vi "VideoRecorderOI.vi"() -> ()   [LabVIEW 2011]
uses:
  <instrlib>/niHWS/nihws.llb/niHWS Open File Permissions ID.ctl
  <vilib>/DAQmx/read.llb/DAQmx Read (Analog 1D Wfm NChan NSamp).vi
  <vilib>/DAQmx/create/channels.llb/DAQmx Create Channel (AI-Voltage-Basic).vi
  <vilib>/DAQmx/configure/timing.llb/DAQmx Timing (Sample Clock).vi
  <vilib>/DAQmx/miscellaneous.llb/DAQmx Fill In Error Info.vi
  <instrlib>/niHWS/nihws.llb/niHWS Write Analog WDT.vi
  <instrlib>/niHWS/nihws.llb/niHWS Write Analog DBL.vi
  <vilib>/vision/driver/NI_Vision_Acquisition_Software.lvlib
  C:/Program Files/National Instruments/LabVIEW 2011/resource/objmgr/imaqdx.rc
  <vilib>/ptbypt/NI_PtbyPt.lvlib
  C:/Program Files/National Instruments/LabVIEW 2011/resource/objmgr/daqmx.rc
  <vilib>/vision/NI_Vision_Development_Module.lvlib
panel:
  in  "?":enum32{"Settings", "Monitor"}(tab)
  in  "Phtd":bool=TRUE
  in  "% Quality":i32=-1
  in  "Selected Path for AVI":path
  in  "Compressor":string(combo)="DV Video Encoder"
  in  "Video Modes":string(combo)="1280x1024 RGB8 10.00fps"
  in  "Camera":string(combo)="uc480 Capture Device 1"
  in  "Recording channels":tag
  in  "Channel Names":string[](array[string])
  in  "reduce size":bool
  in  "Downsampling factor":i32=15
  in  "VISA resource name":refnum<visa-resource-name>
  in  "DPI":dbl=3500.0
  in  "Video":bool=TRUE
  in  "Ephys":bool
  in  "Mouse":bool=TRUE
  in  "Start":bool
  out "Eye camera":T1(plugin-control)
  out "Ephys Recoding Signals":waveform(dbl)[](graph)
  out "Activity":dbl(graph)
  in  "stop":bool
  out "Rec Time":dbl format="%#_3g"
  in  "Display":bool
  out "fps":dbl format="%#_2g"
  in  "Rec":bool
  # "File settings"
  # "Ephys Channels"
  # "Camera settings"
  # "Mouse"
  # "On"
  # "Off"
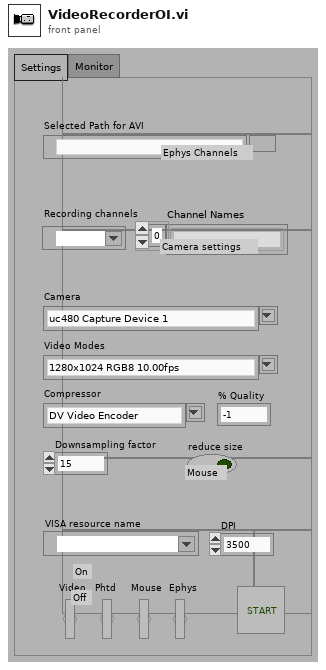
[diagram p1: front panel]
types:
  T1 = typedef "IMAQ Image.ctl" = refnum<image>
  T2 = typedef "niHWS Open File Permissions ID.ctl" = enum32{"Read Only", "Read/Write Existing", "Read/Write/Create New", "Read/Write/Create New Always"}
  T3 = cluster{"Type":u32, "Version":u32, "Flags":u32, "SerialNumberHigh":u32, "SerialNumberLow":u32, "BusType":u32, "InterfaceName":string, "VendorName":string, "ModelName":string, "CameraFileName":string, "CameraAttributeURL":string}[]
  T4 = cluster{"Type":u32, "Version":u32, "Flags":u32, "SerialNumberHigh":u32, "SerialNumberLow":u32, "BusType":u32, "InterfaceName":string, "VendorName":string, "ModelName":string, "CameraFileName":string, "CameraAttributeURL":string}
  T5 = typedef "IMAQdx.ctl" = refnum<k21>
  T6 = cluster{"Video Mode":u32, "Video Mode Name":string}[]
  T7 = typedef "AviRefnum.ctl" = refnum<k1>
  T8 = typedef "Image Type" = u32
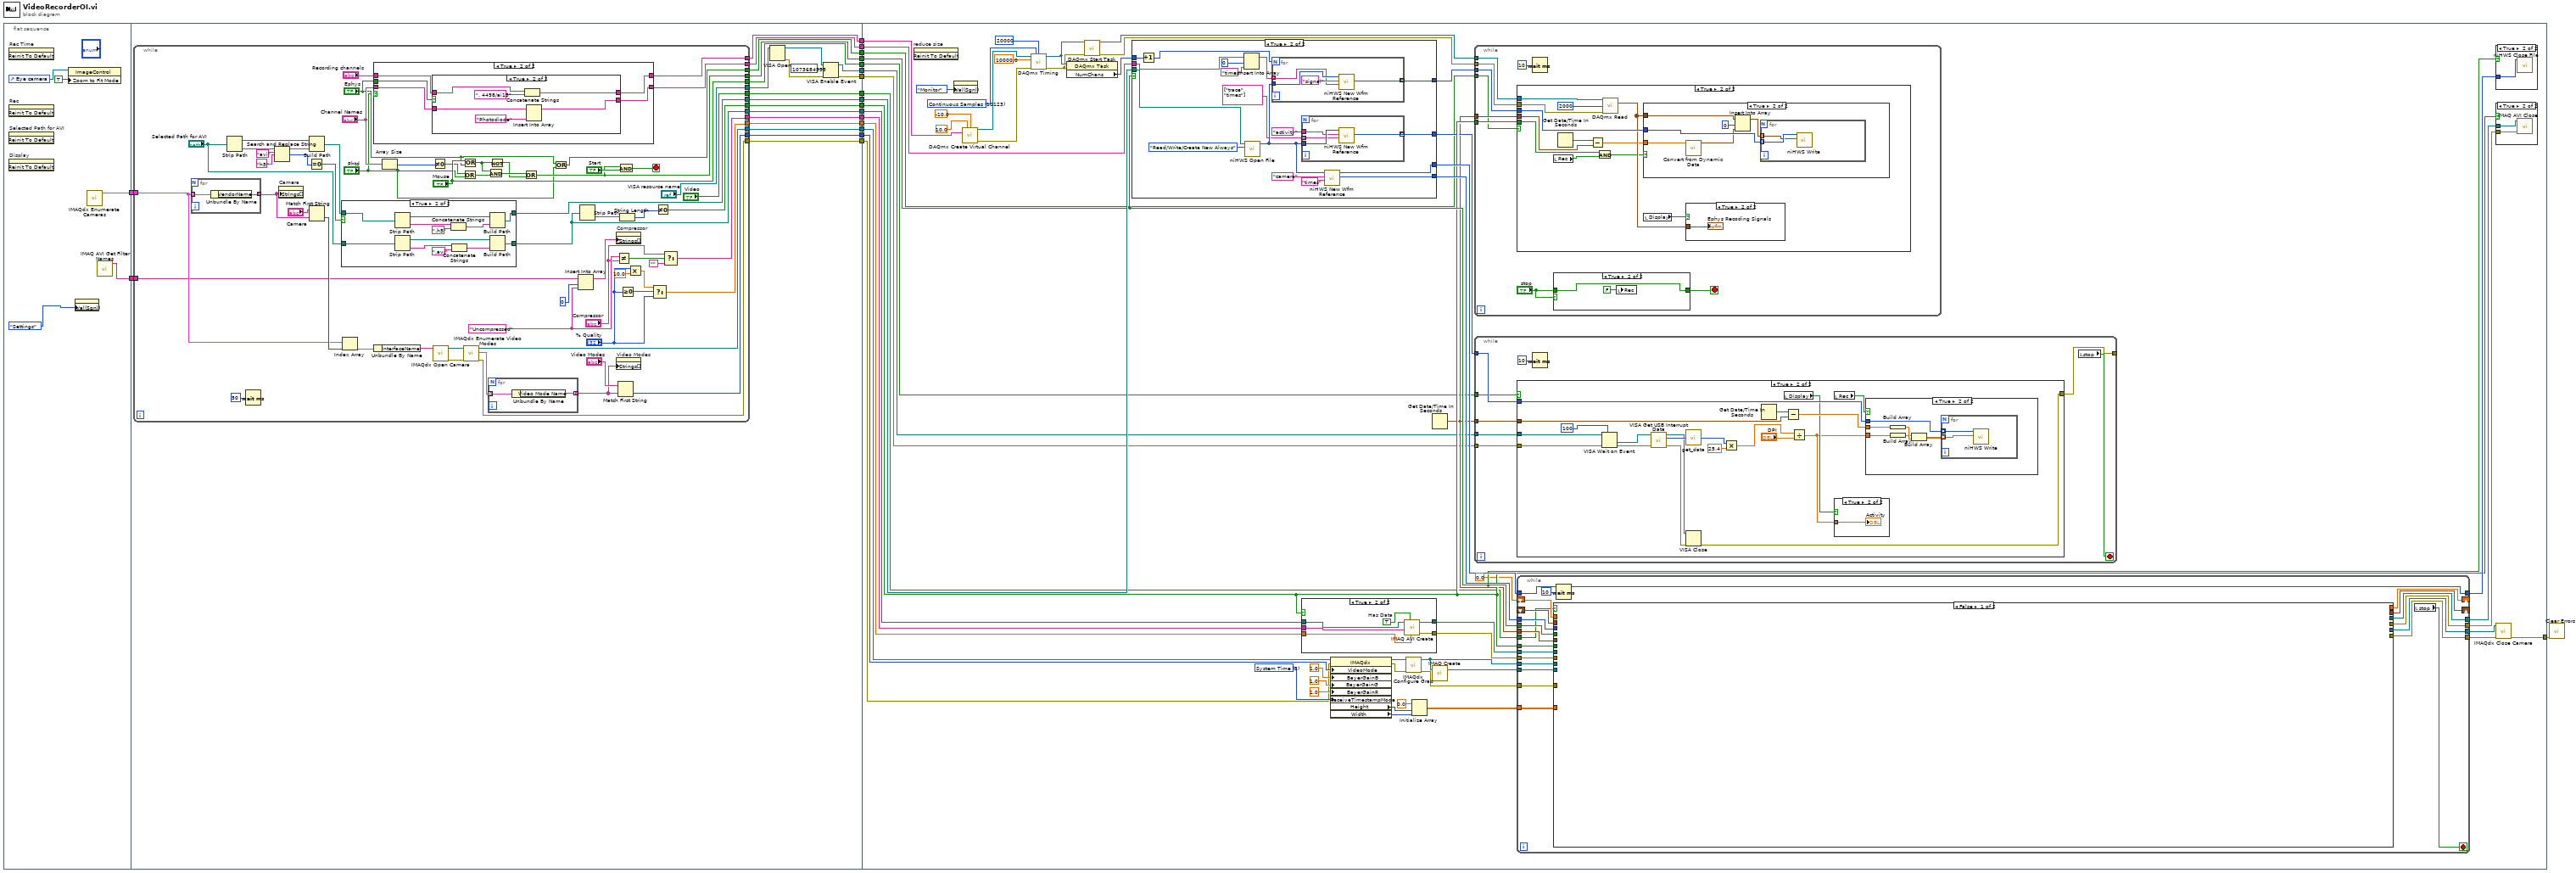
[diagram p0: block diagram]
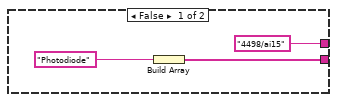
[diagram p3: hidden frame]
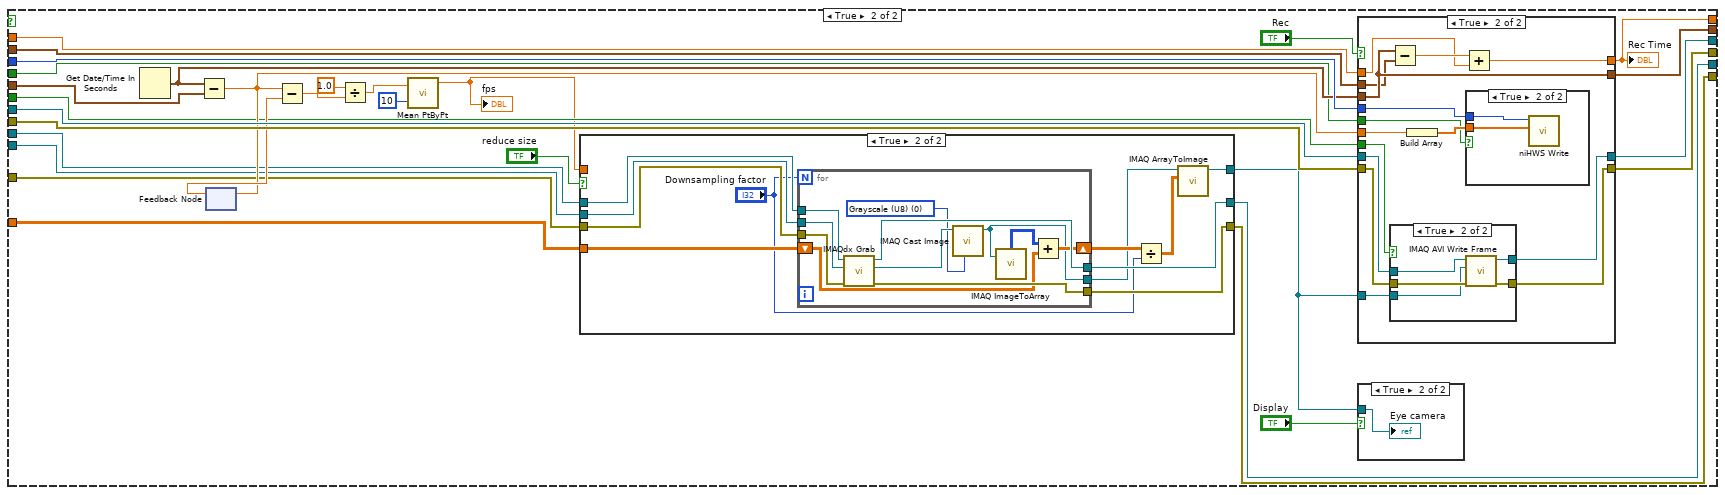
[diagram p16: hidden frame]
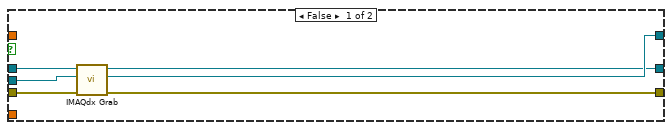
[diagram p17: hidden frame]
diagram:
  n1 = flat-sequence {
    tunnel: [w21] -> w2
    tunnel: [w20] -> w1
    tunnel: [w46] -> w19
    tunnel: [w45] -> w18
    tunnel: [w44] -> w17
    tunnel: [w43] -> w16
    tunnel: [w42] -> w15
    tunnel: [w41] -> w14
    tunnel: [w40] -> w13
    tunnel: [w39] -> w12
    tunnel: [w38] -> w11
    tunnel: [w37] -> w10
    tunnel: [w36] -> w9
    tunnel: [w31] -> w8
    tunnel: [w30] -> w7
    tunnel: [w29] -> w5
    tunnel: [w28] -> w4
    tunnel: [w27] -> w3
    tunnel: w2 -> [w26]
    tunnel: w1 -> [w25]
    tunnel: w19 -> [w186]
    tunnel: w18 -> [w182]
    tunnel: w17 -> [w185]
    tunnel: w16 -> [w184]
    tunnel: w15 -> [w175]
    tunnel: w14 -> [w180]
    tunnel: w13 -> [w176]
    tunnel: w12 -> [w174]
    tunnel: w11 -> [w159]
    tunnel: w10 -> [w143]
    tunnel: w9 -> [w163]
    tunnel: w8 -> [w149]
    tunnel: w7 -> [w148]
    tunnel: [w147] -> w6
    tunnel: w5 -> [w146]
    tunnel: w4 -> [w145]
    tunnel: w3 -> [w144]
    frame #0 {
      n2 = invoke on="Rec Time" class="DigNum (strict)" method="Reinit To Default"() -> ()  [unwired: 3 in, 3 out]
      n3 = control-ref of="Eye camera"() -> (w24:refnum<vi>)
      n4 = invoke on="Rec" class="Bool (strict)" method="Reinit To Default"() -> ()  [unwired: 3 in, 3 out]
      n5 = invoke on="Selected Path for AVI" class="Path" method="Reinit To Default"() -> ()  [unwired: 3 in, 3 out]
      n6 = invoke on="Display" class="Bool (strict)" method="Reinit To Default"() -> ()  [unwired: 3 in, 3 out]
      n7 = property on="Property Node" class="ImageControl"(reference=w24, "Zoom to Fit Mode"=TRUE) -> ()  [unwired: 1 in, 2 out]
      n8 = property class="TabCtl (strict)"("Val(Sgnl)"=enum32{"Settings", "Monitor"}."Settings" ("Value (Signaling)")) -> ()  [unwired: 2 in, 2 out]
      n9 = call <vilib>:"IMAQdx Enumerate Cameras.vi"() -> ("Camera Information Array"=w21:T3)  [unwired: 10 in, 1 out]
      n10 = call "IMAQ AVI Get Filter Names"() -> ("Filter Names"=w20:string[])  [unwired: 10 in, 1 out]
    }
    frame #1 {
      n11 = while {
        tunnel: [w89] -> w46
        tunnel: [w102] -> w45
        tunnel: [w79] -> w44
        tunnel: [w95] -> w43
        tunnel: [w70] -> w42
        tunnel: [w73] -> w41
        tunnel: [w88] -> w40
        tunnel: [w59] -> w39
        tunnel: [w69] -> w38
        tunnel: [w55] -> w37
        tunnel: [w57] -> w36
        tunnel: ["VISA resource name"] -> w32
        tunnel: [w52] -> w29
        tunnel: ["Mouse"] -> w28
        tunnel: ["Video"] -> w27
        tunnel: w26 -> [w48]
        tunnel: w25 -> [w47]
        stop <- w66 stop-if-true
        w100 = "Uncompressed"
        n12 = for {
          tunnel: w48 -> [w139] mode=indexing
          tunnel: [w138] -> w94 mode=indexing
          n13 = Unbundle By Name(w139) -> ("VendorName"=w138:string)
        }
        n14 = Strip Path(path="Selected Path for AVI") -> (stripped path=w87:path, name=w85:string)
        n15 = Wait (ms)(milliseconds to wait=u32 50) -> ()  [unwired: 1 out]
        n16 = Search and Replace String(input string=w85, search string="avi", replace string="h5" ("replace string (\"\")")) -> (result string=w86:string, number of replacements=w76:i32)  [unwired: 5 in, 2 out]
        n17 = property on="Camera" class="CmbBox"("Strings[]"=w94) -> ()  [unwired: 2 in, 2 out]
        n18 = Equal To 0?(x=w76) -> (x = 0?=w75:bool)
        n19 = Build Path(base path=w87, name or relative path=w86) -> (appended path=w74:path)
        n20 = Match First String(2:w94, 3:"Camera") -> (0:w92:i32)  [unwired: 1 out]
        n21 = case shown="True" w75 {
          tunnel: "Selected Path for AVI" -> [w124 w137]
          tunnel: [w124 w136] -> w70
          tunnel: w74 -> [w125 w127]
          tunnel: [w125 w126] -> w73
          frame False {
          }
          frame True {
            n22 = Strip Path(path=w127) -> (stripped path=w131:path, name=w129:string)
            n23 = Strip Path(path=w137) -> (stripped path=w135:path, name=w133:string)
            n24 = Concatenate Strings(w129, ".h5" ("search string")) -> (w128:string)
            n25 = Concatenate Strings(w133, ".avi" ("search string")) -> (w132:string)
            n26 = Build Path(base path=w131, name or relative path=w128) -> (appended path=w126:path)
            n27 = Build Path(base path=w135, name or relative path=w132) -> (appended path=w136:path)
          }
        }
        n28 = Index Array(array=w48, index=w92) -> (element=w91:T4)
        n29 = case shown="True" "Phtd" {
          tunnel: "Channel Names" -> [w109 w113]
          tunnel: [w109 w112] -> w57
          tunnel: "Recording channels" -> [w108 w111]
          tunnel: [w108 w114] -> w55
          tunnel: "Ephys" -> [_ w110]
          frame False {
          }
          frame True {
            n30 = case shown="True" w110 {
              tunnel: ["4498/ai15" w123] -> w114
              tunnel: w113 -> [_ w122]
              tunnel: [w115 w120] -> w112
              tunnel: w111 -> [_ w118]
              frame False {
                n31 = Build Array("Photodiode" ("new element/subarray")) -> (w115:string[])
              }
              frame True {
                n32 = Concatenate Strings(w118, ", 4498/ai15") -> (w123:string)
                n33 = Insert Into Array(array=w122, new element="Photodiode" ("new element/subarray")) -> (w120:string[])  [unwired: 1 in]
              }
            }
          }
        }
        n34 = Unbundle By Name(w91) -> ("InterfaceName"=w90:string)
        n35 = Array Size(array="Channel Names") -> (size(s)=w68:i32)
        n36 = Not Equal To 0?(x=w68) -> (x != 0?=w54:bool)
        n37 = call <vilib>:"IMAQdx Open Camera.vi"("Session In"=w90) -> ("error out"=w106:errorcluster, "Session Out"=w107:T5)  [unwired: 9 in]
        n38 = Or(x=w54, y="Phtd") -> (x .or. y?=w53:bool)
        n39 = Or(x="Mouse", y="Ephys") -> (x .or. y?=w61:bool)
        n40 = call <vilib>:"IMAQdx Enumerate Video Modes.vi"("error in"=w106, "Session In"=w107) -> ("error out"=w88:errorcluster, "Video Modes"=w103:T6, "Session Out"=w89:T5)  [unwired: 6 in, 1 out]
        n41 = And(x=w61, y=w53) -> (x .and. y?=w62:bool)
        n42 = for {
          tunnel: w103 -> [w141] mode=indexing
          tunnel: [w140] -> w96 mode=indexing
          n43 = Unbundle By Name(w141) -> ("Video Mode Name"=w140:string)
        }
        n44 = Not(x=w61) -> (.not. x?=w60:bool)
        n45 = Or(x=w62, y=w60) -> (x .or. y?=w59:bool)
        n46 = Or(x="Ephys", y="Phtd") -> (x .or. y?=w52:bool)
        n47 = Insert Into Array(array=w47, index=0 ("Index"), new element=w100) -> (w104:string[])
        n48 = Strip Path(path=w70) -> (name=w71:string)  [unwired: 1 out]
        n49 = property on="Compressor" class="CmbBox"("Strings[]"=w104) -> ()  [unwired: 2 in, 2 out]
        n50 = Not Equal?(x=w100, y="Compressor") -> (x != y?=w98:bool)
        n51 = property on="Video Modes" class="CmbBox"("Strings[]"=w96) -> ()  [unwired: 2 in, 2 out]
        n52 = Match First String(2:w96, 3:"Video Modes") -> (0:w95:i32)  [unwired: 1 out]
        n53 = And(x=w59, y="Start") -> (x .and. y?=w66:bool)
        n54 = String Length(string=w71) -> (length=w72:i32)
        n55 = Greater Or Equal To 0?(x="% Quality") -> (x >= 0?=w81:bool)
        n56 = Multiply(x="% Quality", y=10.0) -> (x*y=w82:dbl)
        n57 = Select(t=w82, s=w81, f="% Quality") -> (s? t:f=w79:dbl)
        n58 = Not Equal To 0?(x=w72) -> (x != 0?=w69:bool)
        n59 = Select(t="Compressor", s=w98, f="") -> (s? t:f=w102:string)
      }
      n60 = VISA Open(VISA resource name=w32) -> (VISA resource name=w33:refnum<visa-resource-name>, error out=w34:errorcluster)  [unwired: 1 in, 3 out]
      n61 = VISA Enable Event(8:w34, 10:u32 1073684535 ("event type"), 11:w33) -> (0:w30:errorcluster, 3:w31:refnum<visa-resource-name>)  [unwired: 1 out]
    }
    frame #2 {
      w169 = 10123 items=["Finite Samples"=10178, "Continuous Samples"=10123, "Hardware Timed Single Point"=12522] ("sample mode")
      w181 = u32 2 items=["None", "Tick Count", "System Time"] ("ReceiveTimestampMode")
      n62 = invoke on="reduce size" class="Bool (strict)" method="Reinit To Default"() -> ()  [unwired: 3 in, 3 out]
      n63 = property class="TabCtl (strict)"("Val(Sgnl)"=enum32{"Settings", "Monitor"}."Monitor" ("Value (Signaling)")) -> ()  [unwired: 2 in, 2 out]
      n64 = call-poly <vilib>:"DAQmx Create Virtual Channel.vi"("maximum value"=10.0, "minimum value"=-10.0, "physical channels"=w143) -> ("task out"=w170:refnum<k21>, "error out"=w167:errorcluster)  [unwired: 11 in]
      n65 = call-poly <vilib>:"DAQmx Timing.vi"("task/channels in"=w170, "sample mode"=w169, "samples per channel"=20000, "rate"=10000.0, "error in"=w167) -> ("task out"=w162:refnum<k21>, "error out"=w161:errorcluster)  [unwired: 9 in]
      n66 = property class="DAQmx Task"(reference=w162, error in=w161) -> ("NumChans"=w160:u32)  [unwired: 2 out]
      n67 = call <vilib>:"DAQmx Start Task.vi"("task/channels in"=w162, "error in"=w161) -> ("task out"=w165:refnum<k21>, "error out"=w164:errorcluster)  [unwired: 12 in]
      n68 = case shown="True" w174 {
        tunnel: w180 -> [_ w290]
        tunnel: [_ w289] -> w179
        tunnel: [_ w288] -> w178
        tunnel: [_ w287] -> w173
        tunnel: w163 -> [_ w286]
        tunnel: w160 -> [_ w282]
        tunnel: [_ w279] -> w151
        frame False {
        }
        frame True {
          n69 = Increment(x=w282) -> (x+1=w281:u32)
          n70 = Insert Into Array(array=w286, index=0, new element="times" ("group name (empty)")) -> (w283:string[])
          n71 = call <instrlib>:"niHWS Open File.vi"("permissions (0:read only)"=niHWS_Open_File_Permissions_ID."Read/Write/Create New Always", "file path"=w290) -> ("file handle"=w280:u32)  [unwired: 8 in, 1 out]
          n72 = for {
            N: w281 -> [_]
            tunnel: w280 -> [w300]
            tunnel: [w299] -> w287 mode=indexing
            tunnel: w283 -> [w298] mode=indexing
            n73 = call <instrlib>:"niHWS New Wfm Reference.vi"("waveform name (empty)"=w298, "group name (empty)"="signal", "file handle in"=w300) -> ("waveform reference"=w299:u32)  [unwired: 6 in, 2 out]
          }
          n74 = for {
            tunnel: w280 -> [w297]
            tunnel: [w296] -> w279 mode=indexing
            tunnel: "activity" ("group name (empty)") -> [w295]
            tunnel: string[] ["trace", "times"] -> [w294] mode=indexing
            n75 = call <instrlib>:"niHWS New Wfm Reference.vi"("waveform name (empty)"=w294, "group name (empty)"=w295, "file handle in"=w297) -> ("waveform reference"=w296:u32)  [unwired: 6 in, 2 out]
          }
          n76 = call <instrlib>:"niHWS New Wfm Reference.vi"("waveform name (empty)"="times" ("group name (empty)"), "group name (empty)"="camera", "file handle in"=w280) -> ("waveform reference"=w289:u32, "file handle out"=w288:u32)  [unwired: 6 in, 1 out]
        }
      }
      n77 = case shown="True" w159 {
        tunnel: [_ w274] -> w197
        tunnel: [_ w273] -> w194
        tunnel: w185 -> [_ w272]
        tunnel: w182 -> [_ w271]
        tunnel: w175 -> [_ w270]
        frame False {
        }
        frame True {
          w275 = TRUE  # Has Data
          n78 = call "IMAQ AVI Create"("quality"=w272, "Has Data"=w275, "Compression Filter"=w271, "AVI Path"=w270) -> ("error out"=w273:errorcluster, "Avi Refnum"=w274:T7)  [unwired: 3 in, 3 out]
        }
      }
      n79 = property class="IMAQdx"(reference=w186, error in=w176, "VideoMode"=w184, "BayerGainB"=1.0, "BayerGainG"=1.0, "BayerGainR"=1.0, "ReceiveTimestampMode"=w181) -> (reference out=w188:T5, error out=w187:errorcluster, "Height"=w157:u32, "Width"=w156:u32)
      n80 = call <vilib>:"IMAQdx Configure Grab.vi"("error in"=w187, "Session In"=w188) -> ("error out"=w192:errorcluster, "Session Out"=w183:T5)  [unwired: 8 in]
      n81 = Initialize Array(0.0 ("element"), w157, w156) -> (w155:dbl[][])
      n82 = Get Date/Time In Seconds() -> (seconds since 1Jan1904=w150:timestamp)
      n83 = call "IMAQ Create"("Image Name"=w183) -> ("New Image"=w193:T1)  [unwired: 4 in, 1 out]
      n84 = while {
        tunnel: w173 -> [w243]
        tunnel: w165 -> [w242]
        tunnel: w164 -> [w241]
        tunnel: w150 -> [w240]
        tunnel: w159 -> [w238]
        tunnel: w146 -> [w235]
        stop <- w236 stop-if-true
        n85 = case shown="True" w235 {
          tunnel: w243 -> [_ w255]
          tunnel: w242 -> [_ w253]
          tunnel: w241 -> [_ w252]
          tunnel: w240 -> [_ w249]
          tunnel: w238 -> [_ w246]
          frame False {
          }
          frame True {
            n86 = local read "Rec"() -> (w245:bool)
            n87 = Get Date/Time In Seconds() -> (seconds since 1Jan1904=w250:timestamp)
            n88 = Subtract(x=w250, y=w249) -> (x-y=w248:dbl)
            n89 = And(x=w246, y=w245) -> (x .and. y?=w244:bool)
            n90 = call-poly <vilib>:"DAQmx Read.vi"("task/channels in"=w253, "number of samples per channel"=2000, "error in"=w252) -> ("data"=w251:waveform(dbl)[])  [unwired: 10 in, 2 out]
            n91 = case shown="True" w244 {
              tunnel: w255 -> [_ w262]
              tunnel: w251 -> [_ w260]
              tunnel: w248 -> [_ w261]
              frame False {
              }
              frame True {
                n92 = call "Convert from Dynamic Data"("Dynamic Data Type"=w261) -> ("Waveform"=w259:waveform(dbl))  [unwired: 3 in]
                n93 = Insert Into Array(array=w260, index=0, new element=w259) -> (w257:waveform(dbl)[])
                n94 = for {
                  tunnel: w262 -> [w264] mode=indexing
                  tunnel: w257 -> [w263] mode=indexing
                  n95 = call-poly <instrlib>:"niHWS Write.vi"("analog waveform"=w263, "waveform reference in"=w264) -> ()  [unwired: 8 in, 2 out]
                }
              }
            }
            n96 = local read "Display"() -> (w247:bool)
            n97 = case shown="True" w247 {
              tunnel: w251 -> [_ w256]
              frame False {
              }
              frame True {
                "Ephys Recoding Signals" <- w256
              }
            }
          }
        }
        n98 = Wait (ms)(milliseconds to wait=u32 10) -> ()  [unwired: 1 out]
        n99 = case shown="True" "stop" {
          tunnel: "stop" -> [w265 w266]
          tunnel: [w265 w266] -> w236
          frame False {
          }
          frame True {
            n100 = local write "Rec"(FALSE ("Rec")) -> ()
          }
        }
      }
      n101 = while {
        tunnel: w151 -> [w203]
        tunnel: w150 -> [w204]
        tunnel: w149 -> [w202]
        tunnel: w148 -> [w201]
        tunnel: [w200] -> _
        tunnel: w145 -> [w199]
        stop <- w205 stop-if-true
        n102 = case shown="True" w199 {
          tunnel: w204 -> [_ w225]
          tunnel: w203 -> [_ w223]
          tunnel: w202 -> [_ w212]
          tunnel: w201 -> [_ w211]
          tunnel: [_ w208] -> w200
          frame False {
          }
          frame True {
            n103 = VISA Wait on Event(7:u32 100 ("timeout (0)"), 8:w211, 11:w212) -> (0:w215:errorcluster, 1:w214:refnum<visa-resource-name>)  [unwired: 4 out]
            n104 = call <vilib>:"VISA Get USB Interrupt Data.vi"("error in (no error)"=w215, "VISA USB Intr Event"=w214) -> ("error out"=w217:errorcluster, "data buffer"=w218:u8[], "VISA USB Intr Event out"=w216:refnum<visa-resource-name>)  [unwired: 7 out]
            n105 = call "get_data.vi"("data buffer"=w218) -> ("X Value"=w206:i8)  [unwired: 2 out]
            n106 = VISA Close(VISA resource name=w216, error in (no error)=w217) -> (error out=w208:errorcluster)
            n107 = Multiply(x=w206, y=25.4) -> (x*y=w221:dbl)
            n108 = Get Date/Time In Seconds() -> (seconds since 1Jan1904=w224:timestamp)
            n109 = local read "Display"() -> (w210:bool)
            n110 = Subtract(x=w224, y=w225) -> (x-y=w222:dbl)
            n111 = Divide(x=w221, y="DPI") -> (x/y=w209:dbl)
            n112 = local read "Rec"() -> (w207:bool)
            n113 = case shown="True" w210 {
              tunnel: w209 -> [_ w226]
              frame False {
              }
              frame True {
                "Activity" <- w226
              }
            }
            n114 = case shown="True" w207 {
              tunnel: w223 -> [_ w232]
              tunnel: w222 -> [_ w231]
              tunnel: w209 -> [_ w227]
              frame False {
              }
              frame True {
                n115 = Build Array(w231) -> (w230:dbl[])
                n116 = Build Array(w227) -> (w228:dbl[])
                n117 = Build Array(w228, w230) -> (w229:dbl[][])
                n118 = for {
                  tunnel: w229 -> [w234] mode=indexing
                  tunnel: w232 -> [w233] mode=indexing
                  n119 = call-poly <instrlib>:"niHWS Write.vi"("data"=w234, "waveform reference in"=w233) -> ()  [unwired: 8 in, 2 out]
                }
              }
            }
          }
        }
        n120 = Wait (ms)(milliseconds to wait=u32 10) -> ()  [unwired: 1 out]
        n121 = local read "stop"() -> (w205:bool)
      }
      n122 = while {
        tunnel: [w323] -> w196
        tunnel: [w322] -> w195
        tunnel: w197 -> [w321]
        tunnel: w194 -> [w320]
        tunnel: w193 -> [w310]
        tunnel: w183 -> [w311]
        tunnel: w192 -> [w309]
        tunnel: w150 -> [w319]
        tunnel: w179 -> [w318]
        tunnel: w178 -> [w317]
        tunnel: [w317] -> w177
        shift-right: [w316] -> _
        shift-left: _ -> [w315]
        tunnel: w174 -> [w313]
        tunnel: w159 -> [w314]
        tunnel: w155 -> [w312]
        tunnel: [w308] -> w154
        tunnel: [w307] -> w153
        shift-right: [w305] -> _
        shift-left: 0.0 -> [w306]
        tunnel: w144 -> [w304]
        stop <- w303 stop-if-true
        n123 = case shown="False" w304 {
          tunnel: [_ w353] -> w323
          tunnel: [_ w352] -> w322
          tunnel: w321 -> [_ w351]
          tunnel: w320 -> [_ w350]
          tunnel: w319 -> [_ w348]
          tunnel: w318 -> [_ w342]
          tunnel: [_ w340] -> w316
          tunnel: w315 -> [_ w339]
          tunnel: w314 -> [_ w337]
          tunnel: w313 -> [_ w336]
          tunnel: w312 -> [_ w333]
          tunnel: w311 -> [_ w332]
          tunnel: w310 -> [_ w331]
          tunnel: w309 -> [_ w330]
          tunnel: [_ w329] -> w308
          tunnel: [_ w328] -> w307
          tunnel: w306 -> [_ w327]
          tunnel: [_ w326] -> w305
          frame False {
          }
          frame True {
            n124 = Get Date/Time In Seconds() -> (seconds since 1Jan1904=w341:timestamp)
            n125 = Subtract(x=w341, y=w348) -> (x-y=w343:dbl)
            n126 = feedback #1() -> (w347:dbl)  [unwired: 1 in]
            n127 = feedback-in #1(w343) -> ()
            n128 = Subtract(x=w343, y=w347) -> (x-y=w345:dbl)
            n129 = Divide(x=1.0, y=w345) -> (x/y=w344:dbl)
            n130 = call <vilib>:"Mean PtByPt.vi"("x"=w344, "sample length"=10) -> ("mean"=w325:dbl)  [unwired: 2 in, 1 out]
            "fps" <- w325
            n131 = case shown="True" "reduce size" {
              tunnel: [w359 w364] -> w335
              tunnel: w325 -> [_ _]
              tunnel: w333 -> [_ w370]
              tunnel: w332 -> [w358 w369]
              tunnel: w331 -> [w357 w368]
              tunnel: w330 -> [w356 w367]
              tunnel: [w354 w366] -> w328
              tunnel: [w355 w365] -> w329
              frame False {
                n132 = call <vilib>:"IMAQdx Grab.vi"("error in"=w356, "Image In"=w357, "Session In"=w358) -> ("error out"=w354:errorcluster, "Image Out"=w359:T1, "Session Out"=w355:T5)  [unwired: 5 in, 1 out]
              }
              frame True {
                n133 = for {
                  N: "Downsampling factor" -> [_]
                  tunnel: w369 -> [w381]
                  tunnel: w368 -> [w380]
                  tunnel: w367 -> [w378]
                  tunnel: [w377] -> w366
                  tunnel: [w376] -> w365
                  shift-right: [w372] -> w363
                  shift-left: w370 -> [w373]
                  tunnel: [w371] -> w361
                  w375 = T8 0 items=["Grayscale (U8)", "Grayscale (I16)", "Grayscale (SGL)", "Complex (CSG)", "RGB (U32)", "HSL (U32)", "RGB (U64)", "Grayscale (U16)"] ("Image Type")
                  n134 = call <vilib>:"IMAQdx Grab.vi"("error in"=w378, "Image In"=w380, "Session In"=w381) -> ("error out"=w377:errorcluster, "Image Out"=w379:T1, "Session Out"=w376:T5)  [unwired: 5 in, 1 out]
                  n135 = call "IMAQ Cast Image"("Image Type"=w375, "Image Src"=w379) -> ("Image Dst Out"=w371:T1)  [unwired: 8 in, 1 out]
                  n136 = call "IMAQ ImageToArray"("Image"=w371) -> ("Image Pixels (U8)"=w374:u8[][])  [unwired: 3 in, 4 out]
                  n137 = Add(x=w374, y=w373) -> (x+y=w372:dbl[][])
                }
                n138 = Divide(x=w363, y="Downsampling factor") -> (x/y=w362:dbl[][])
                n139 = call "IMAQ ArrayToImage"("Image Pixels (U8)"=w362, "Image"=w361) -> ("Image Out"=w364:T1)  [unwired: 8 in, 1 out]
              }
            }
            n140 = case shown="True" "Rec" {
              tunnel: [w384 w400] -> w353
              tunnel: [w385 w399] -> w352
              tunnel: w351 -> [w384 w398]
              tunnel: w350 -> [w385 w397]
              tunnel: w335 -> [_ w396]
              tunnel: [w382 w386] -> w326
              tunnel: w343 -> [_ w395]
              tunnel: w342 -> [_ w393]
              tunnel: [w383 w391] -> w340
              tunnel: w341 -> [w383 w391]
              tunnel: w339 -> [_ w390]
              tunnel: w336 -> [_ w389]
              tunnel: w337 -> [_ w388]
              tunnel: w327 -> [w382 w387]
              frame False {
              }
              frame True {
                n141 = Subtract(x=w391, y=w390) -> (x-y=w392:dbl)
                n142 = case shown="True" w388 {
                  tunnel: [_ w405] -> w400
                  tunnel: [_ w404] -> w399
                  tunnel: w398 -> [_ w403]
                  tunnel: w397 -> [_ w402]
                  tunnel: w396 -> [_ w401]
                  frame False {
                  }
                  frame True {
                    n143 = call "IMAQ AVI Write Frame"("error in (no error)"=w402, "Image"=w401, "Avi Refnum"=w403) -> ("error out"=w404:errorcluster, "Avi Refnum (duplicate)"=w405:T7)  [unwired: 7 in]
                  }
                }
                n144 = Build Array(w395) -> (w394:dbl[])
                n145 = Add(x=w392, y=w387) -> (x+y=w386:dbl)
                n146 = case shown="True" w389 {
                  tunnel: w394 -> [_ w407]
                  tunnel: w393 -> [_ w406]
                  frame False {
                  }
                  frame True {
                    n147 = call-poly <instrlib>:"niHWS Write.vi"("data"=w407, "waveform reference in"=w406) -> ()  [unwired: 8 in, 2 out]
                  }
                }
              }
            }
            "Rec Time" <- w326
            n148 = case shown="True" "Display" {
              tunnel: w335 -> [_ w408]
              frame False {
              }
              frame True {
                "Eye camera" <- w408
              }
            }
          }
        }
        n149 = Wait (ms)(milliseconds to wait=u32 10) -> ()  [unwired: 1 out]
        n150 = local read "stop"() -> (w303:bool)
      }
      n151 = case shown="True" w174 {
        tunnel: w177 -> [_ w276]
        frame False {
        }
        frame True {
          n152 = call <instrlib>:"niHWS Close File.vi"("file handle"=w276) -> ()  [unwired: 10 in, 1 out]
        }
      }
      n153 = case shown="True" w159 {
        tunnel: w196 -> [_ w269]
        tunnel: w195 -> [_ w268]
        frame False {
        }
        frame True {
          n154 = call "IMAQ AVI Close"("error in (no error)"=w268, "Avi Refnum"=w269) -> ()  [unwired: 9 in, 1 out]
        }
      }
      n155 = call <vilib>:"IMAQdx Close Camera.vi"("error in"=w153, "Session In"=w154) -> ("error out"=w147:errorcluster)  [unwired: 9 in]
    }
  }
  n156 = call <vilib>:"Clear Errors.vi"("error in (no error)"=w6) -> ()  [unwired: 6 in, 1 out]
